vi "Write Name.vi"(8 "error in (no error)":errorcluster, 10 "Name":string, 11 "Process Generator In":refnum<class "Process Generator.lvclass">) -> (0 "error out":errorcluster, 3 "Process Generator Out":refnum<class "Process Generator.lvclass">)   [LabVIEW 2020, in "Process Generation.lvlib" / "Process Generator.lvclass"]
uses:
  Process Generator.lvclass
  Process Generator.lvclass/Process Generator.ctl
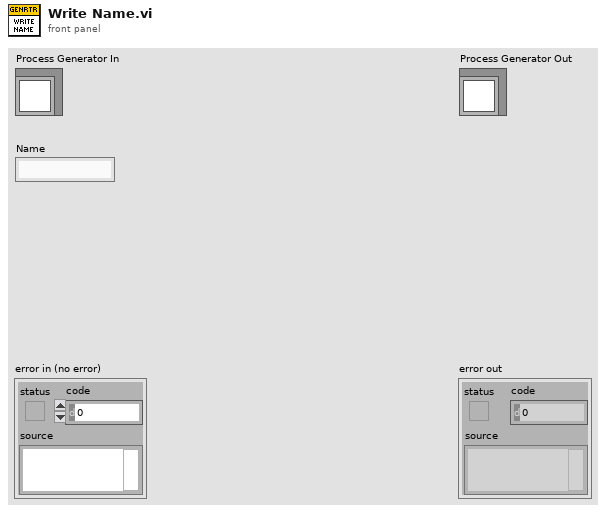
[diagram p1: front panel]
types:
  T1 = typedef "LabVIEW Icon API.lvlib/API_Rectangle Colors.ctl" = cluster{"Border":u32, "Background":u32}
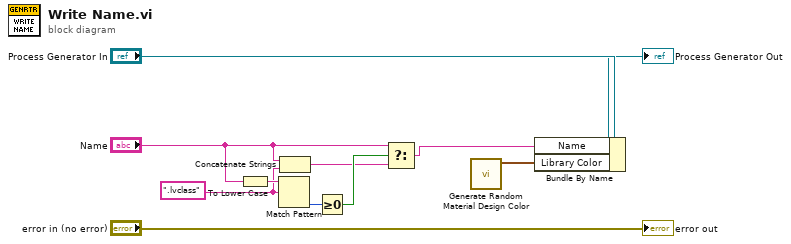
[diagram p0: block diagram]
diagram:
  w4 = ".lvclass"
  n1 = To Lower Case(string="Name") -> (all lower case string=w8:string)
  n2 = Match Pattern(string=w8, regular expression=w4) -> (offset past match=w7:i32)  [unwired: 1 in, 3 out]
  n3 = Concatenate Strings("Name", w4) -> (w2:string)
  n4 = Greater Or Equal To 0?(x=w7) -> (x >= 0?=w6:bool)
  n5 = Select(t="Name", s=w6, f=w2) -> (s? t:f=w5:string)
  n6 = call "Generate Random Material Design Color.vi"() -> ("Random colors"=w1:T1)  [unwired: 11 in]
  n7 = Bundle By Name(cluster="Process Generator In", "Name"=w5, "Library Color"=w1) -> (→"Process Generator Out":refnum<class "Process Generator.lvclass">)
  "error out" <- "error in (no error)"
